vi "Utility.FindNewDataFile.vi"(8 "error in (no error)":errorcluster, 9 "LookupTable":variant, 11 "Parameters":T1={"Results Path"=path "C:/Conti/Logs", "Temp Path"=path "C:/Conti/Temp", "Remote Path"=path "d:/Conti/Logs", "Analysis VIs"=[], "Report Passed?"=FALSE, "Group Channels?"=FALSE}) -> (0 "error out":errorcluster, 1 "LookupTable out":variant, 2 "Found":bool, 3 "Data Path":path)   [LabVIEW 2015, in "NIAnalysis.lvlib"]
uses:
  NIAnalysis.lvlib
  Types/AnalysisGUI.Parameters.ctl
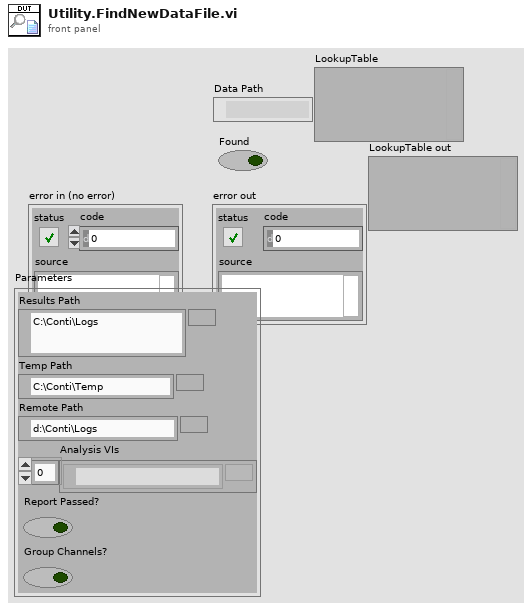
[diagram p1: front panel]
types:
  T1 = typedef "NIAnalysis.lvlib/AnalysisGUI.Parameters.ctl" = cluster{"Results Path":path, "Temp Path":path, "Remote Path":path, "Analysis VIs":path[], "Report Passed?":bool, "Group Channels?":bool}
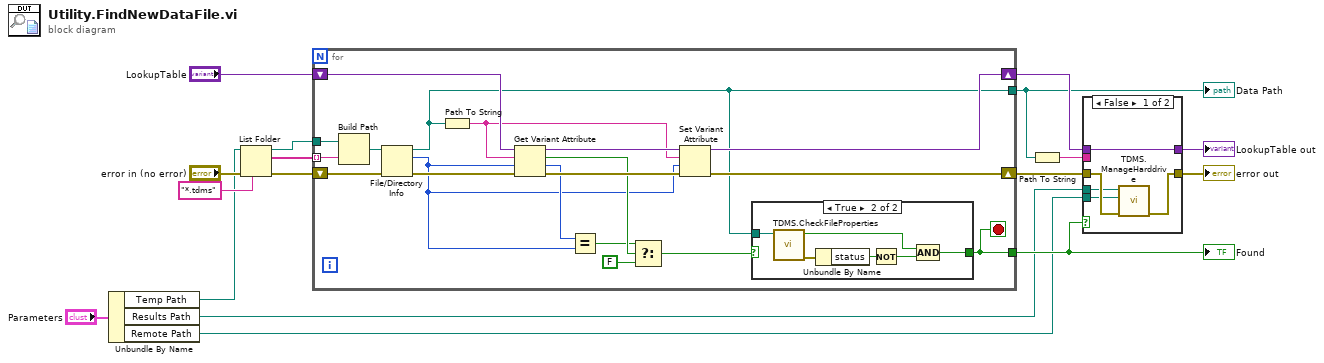
[diagram p0: block diagram]
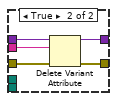
[diagram p2: hidden frame]
diagram:
  n1 = Unbundle By Name("Parameters") -> ("Temp Path"=w1:path, "Results Path"=w3:path, "Remote Path"=w2:path)
  n2 = List Folder(path=w1, pattern="*.tdms", error in="error in (no error)") -> (path out=w13:path, filenames=w14:string[], error out=w15:errorcluster)  [unwired: 1 in, 1 out]
  n3 = for {
    tunnel: w13 -> [w36]
    tunnel: w14 -> [w35] mode=indexing
    shift-right: [w28] -> w11
    shift-left: w15 -> [w34]
    tunnel: [w18] -> w5
    tunnel: [w20] -> w6
    shift-right: [w21] -> w9
    shift-left: "LookupTable" -> [w31]
    stop <- w18 stop-if-true
    n4 = Build Path(base path=w36, name or relative path=w35) -> (appended path=w33:path)
    n5 = File/Directory Info(path=w33, error in=w34) -> (path out=w20:path, size=w24:i64, error out=w32:errorcluster)  [unwired: 4 out]
    n6 = Path To String(path=w20) -> (string=w27:string)
    n7 = Get Variant Attribute(Variant=w31, name=w27, default value (empty Variant)=w24, error in=w32) -> (duplicate Variant=w30:variant, found=w26:bool, value=w25:i64, error out=w29:errorcluster)
    n8 = Equal?(x=w25, y=w24) -> (x = y?=w23:bool)
    n9 = Select(t=w23, s=w26, f=FALSE) -> (s? t:f=w19:bool)
    n10 = Set Variant Attribute(Variant=w30, name=w27, value=w24, error in=w29) -> (Variant out=w21:variant, error out=w28:errorcluster)  [unwired: 1 out]
    n11 = case shown="True" w19 {
      selector: w19 -> [w37 _]
      tunnel: w20 -> [_ w41]
      tunnel: [w37 w39] -> w18
      frame False {
      }
      frame True {
        n12 = call "TDMS.CheckFileProperties.vi"("Data"=w41) -> ("error out"=w40:errorcluster, "Found All"=w38:bool)  [unwired: 9 in]
        n13 = Unbundle By Name(w40) -> ("status"=w43:bool)
        n14 = Not(x=w43) -> (.not. x?=w42:bool)
        n15 = Compound Arithmetic op=AND(w38, w42) -> (w39:bool)
      }
    }
  }
  "Data Path" <- w6
  "Found" <- w5
  n16 = Path To String(path=w6) -> (string=w7:string)
  n17 = case shown="False" w5 {
    tunnel: w11 -> [w47 w53]
    tunnel: [w46 w52] -> w10
    tunnel: w9 -> [w48 w51]
    tunnel: [w48 w50] -> w8
    tunnel: w7 -> [_ w49]
    tunnel: w3 -> [w45 _]
    tunnel: w2 -> [w44 _]
    frame False {
      n18 = call "TDMS.ManageHarddrive.vi"("error in"=w47, "Remote Path"=w44, "Results Path"=w45) -> ("error out"=w46:errorcluster)  [unwired: 8 in]
    }
    frame True {
      n19 = Delete Variant Attribute(4:w53, 6:w49, 7:w51) -> (0:w52:errorcluster, 3:w50:variant)  [unwired: 1 out]
    }
  }
  "error out" <- w10
  "LookupTable out" <- w8
